vi "SetVelocity.vi"(8 "Error In":errorcluster, 10 "Velocity":dbl, 11 "Thorlabs In":refnum<class "Thorlabs.lvclass">) -> (0 "Error Out":errorcluster, 3 "Thorlabs Out":refnum<class "Thorlabs.lvclass">)   [LabVIEW 2018, in "Thorlabs.lvlib" / "Thorlabs.lvclass"]
doc: "This VI sets the Max Velocity on the device when it moves.\n\nCreator: Slade Jeppesen\nCreated Date: 09/29/20"
uses:
  Thorlabs.lvclass
  Thorlabs.lvclass/Thorlabs.ctl
  C:/AME Test Engineering/LabVIEW/PPLs/Axis/DLLs/ThorLabs.MotionControl.KCube.DCServoCLI.dll
  PPLs/Axis/DLLs/ThorLabs.MotionControl.KCube.DCServoCLI.dll
  C:/AME Test Engineering/LabVIEW/PPLs/Axis/DLLs/Thorlabs.MotionControl.GenericMotorCLI.dll
  PPLs/Axis/DLLs/Thorlabs.MotionControl.GenericMotorCLI.dll
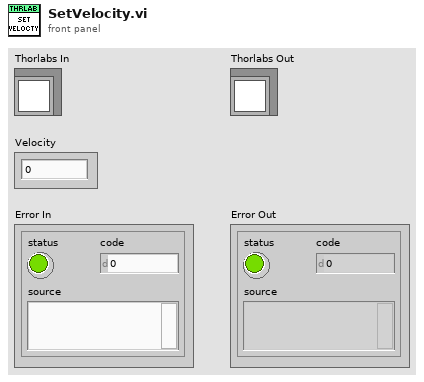
[diagram p1: front panel]
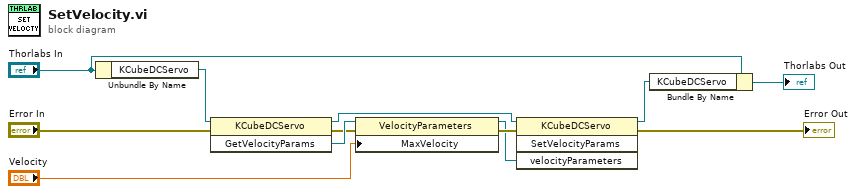
[diagram p0: block diagram]
diagram:
  n1 = Unbundle By Name("Thorlabs In") -> ("KCubeDCServo"=w12:refnum<k24>)
  n2 = invoke class="KCubeDCServo" method="GetVelocityParams"(reference=w12, error in="Error In") -> (reference out=w8:refnum<k24>, error out=w10:errorcluster, "GetVelocityParams"=w11:refnum<k24>)  [unwired: 1 in]
  n3 = property class="VelocityParameters"(reference=w11, error in=w10, "MaxVelocity"="Velocity") -> (reference out=w7:refnum<k24>, error out=w9:errorcluster)
  n4 = invoke class="KCubeDCServo" method="SetVelocityParams"(reference=w8, error in=w9, "velocityParameters"=w7) -> (reference out=w4:refnum<k24>, error out=→"Error Out":errorcluster)  [unwired: 1 in, 2 out]
  n5 = Bundle By Name(cluster="Thorlabs In", "KCubeDCServo"=w4) -> (→"Thorlabs Out":refnum<class "Thorlabs.lvclass">)
